vi "Read Live Trav position.vi"() -> ()   [LabVIEW 2021]
uses:
  <vilib>/BioRobotics/Sensor Drivers/OptiTrack Motive/Controls/OptiTrack_Comm Server Data.ctl
  <vilib>/BioRobotics/Sensor Drivers/OptiTrack Motive/Controls/OptiTrack_Parameters.ctl
  <vilib>/BioRobotics/Sensor Drivers/OptiTrack Motive/Controls/OptiTrack_Frame Data.ctl
  <vilib>/BioRobotics/Sensor Drivers/OptiTrack Motive/Controls/OptiTrack_Comm FGV Action.ctl
  <vilib>/Utility/miscctls.llb/LVPointTypeDef.ctl
  ADAM Client/Sub VIs/ADAM Controls/Update_scan_value.ctl
  Optitrack Global.vi
  <vilib>/BioRobotics/Sensor Drivers/OptiTrack Motive/OptiTrack Motive.lvlib
  <vilib>/BioRobotics/Common Tools/BioRobotics Common Tools.lvlib
  <vilib>/Analysis/NI_AALBase.lvlib
panel:
  in  "Teach Position X,Y,Z,":sgl[](array[numeric])
  in  "Set Position to":bool
  in  "Averaging":i32=30
  out "X,Y,Z, Rx, Ry, Rz":sgl[](array[numeric])
  out "OptiTrack Data":T1
  in  "stop":bool
  out "Streaming Server Running":bool
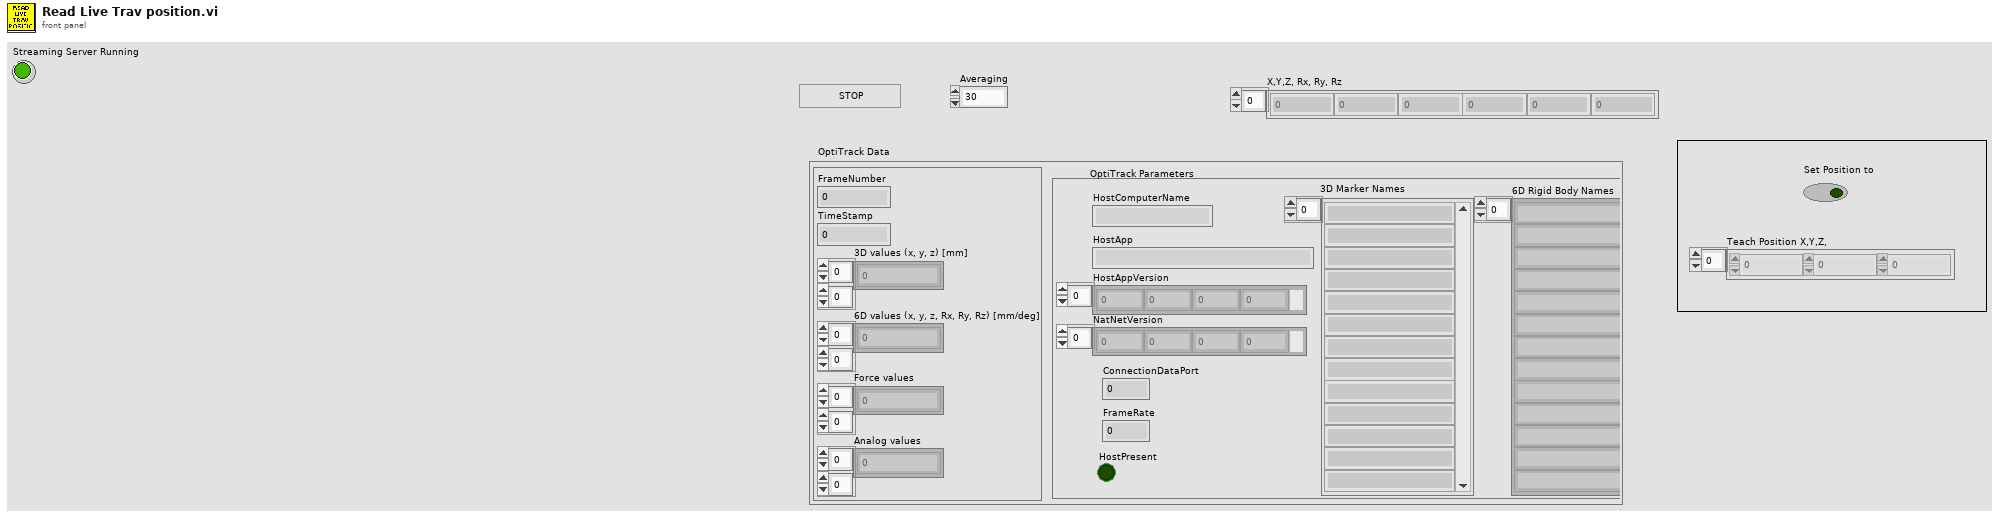
[diagram p1: front panel]
types:
  T1 = typedef "OptiTrack Motive.lvlib/OptiTrack_Comm Server Data.ctl" = cluster{"OptiTrack Parameters":T2, "OptiTrack Frame Data":T3}
  T2 = typedef "OptiTrack Motive.lvlib/OptiTrack_Parameters.ctl" = cluster{"HostComputerName":string, "HostApp":string, "HostAppVersion":u8[], "NatNetVersion":u8[], "ConnectionDataPort":u16, "HostPresent":bool, "3D Marker Names":string[], "6D Rigid Body Names":string[], "Skeletons":string[], "Force Plate Channel Names":string[], "Analog Channel Names":string[], "FrameRate":sgl}
  T3 = typedef "OptiTrack Motive.lvlib/OptiTrack_Frame Data.ctl" = cluster{"FrameNumber":i32, "TimeStamp":i64, "3D values (x, y, z) [mm]":sgl[][], "6D values (x, y, z, Rx, Ry, Rz) [mm/deg]":sgl[][], "Force values":sgl[][], "Analog values":sgl[][]}
  T4 = typedef "LVPointTypeDef.ctl" = cluster{"Horizontal":i16, "Vertical":i16}
  T5 = typedef "OptiTrack Motive.lvlib/OptiTrack_Comm FGV Action.ctl" = enum16{"Initialize", "Set Ethernet Settings", "Read All Data", "Set Parameters", "Start Streaming Server", "Stop Streaming Server", "Set Streaming Data", "Get Streaming Data", "Save Configuration", "Load Configuration", "Connect", "Disconnect", "Streaming Server Running", "Get Data"}
  T6 = typedef "Update_scan_value.ctl" = cluster{"Channel Name":string, "New Value":dbl, "!Auto_Off":bool}
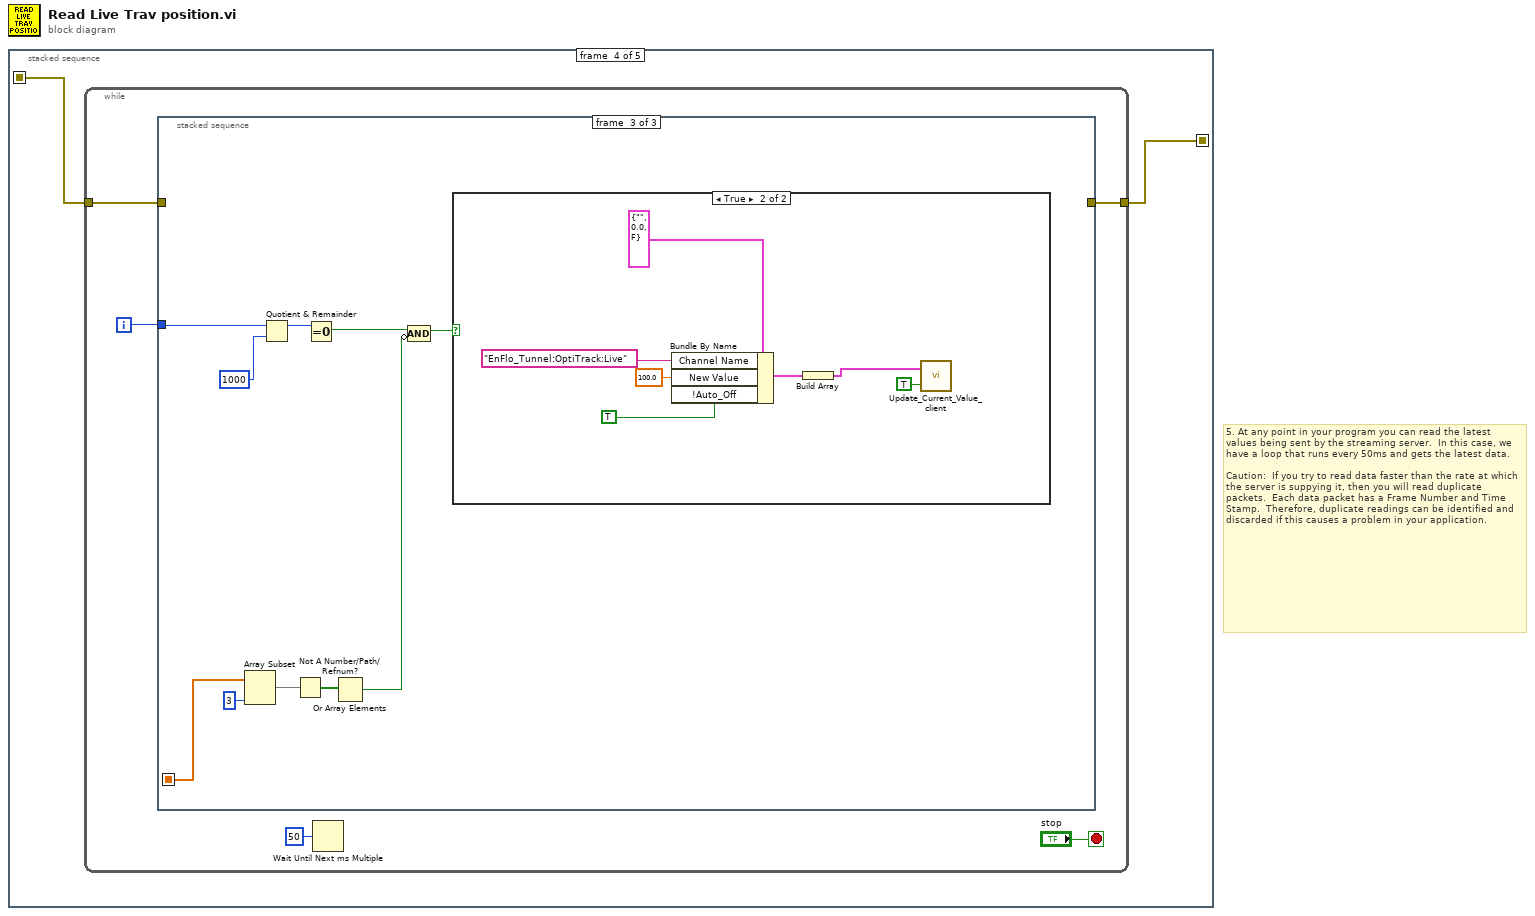
[diagram p0: block diagram]
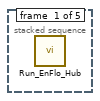
[diagram p2: hidden frame]
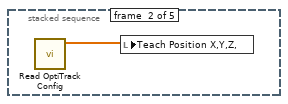
[diagram p3: hidden frame]
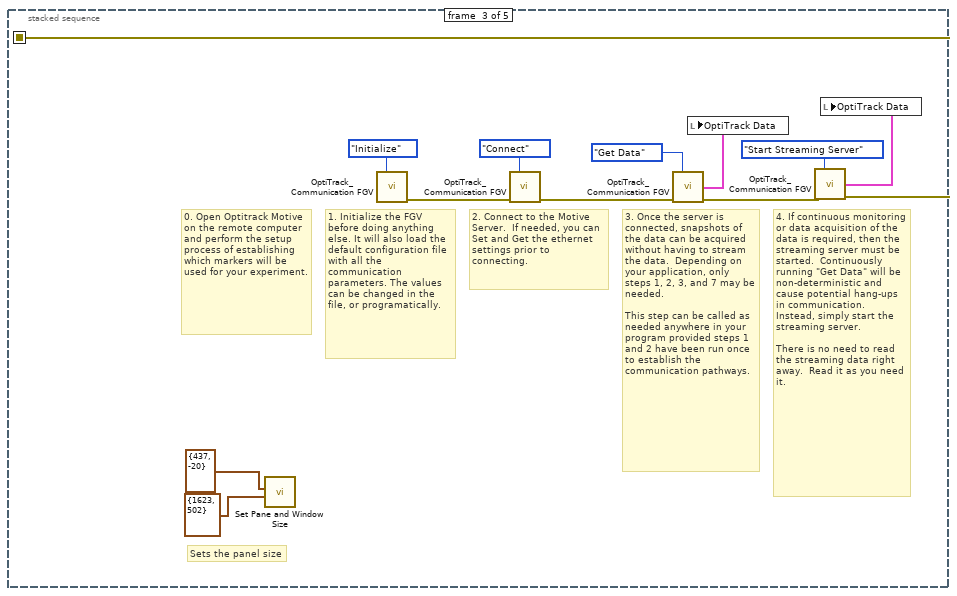
[diagram p4: hidden frame]
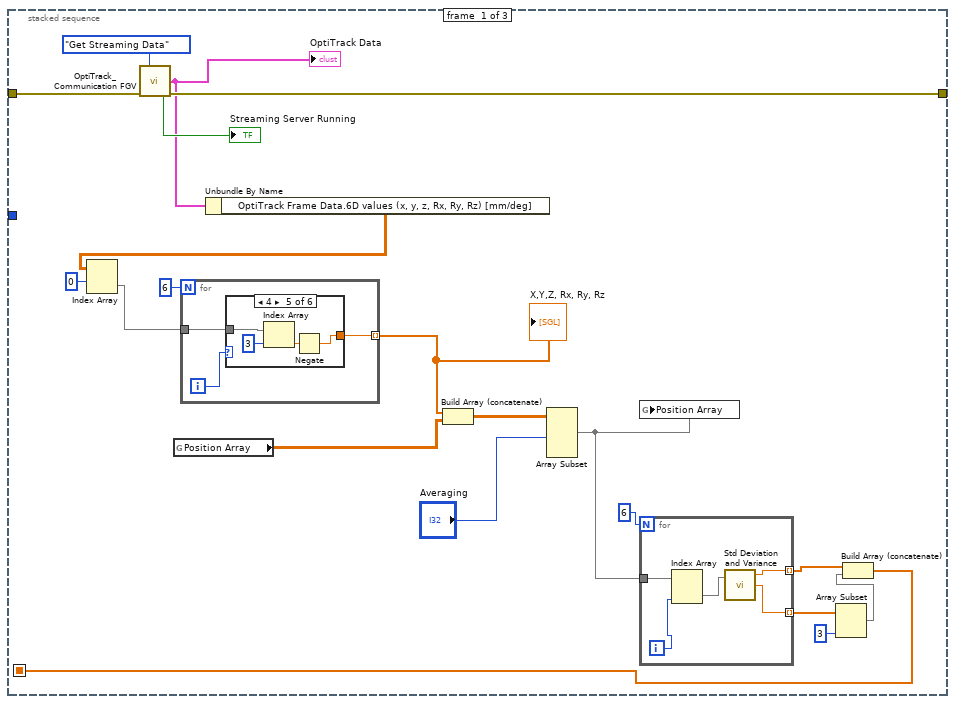
[diagram p5: hidden frame]
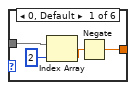
[diagram p6: hidden frame]
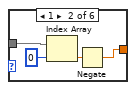
[diagram p7: hidden frame]
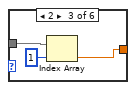
[diagram p8: hidden frame]
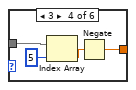
[diagram p9: hidden frame]
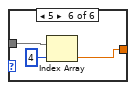
[diagram p10: hidden frame]
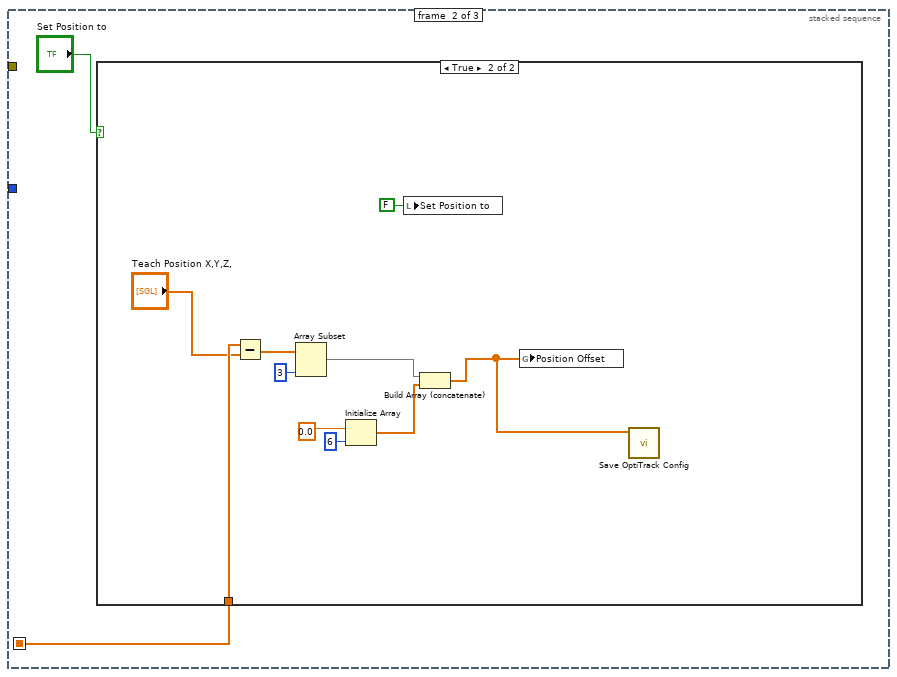
[diagram p11: hidden frame]
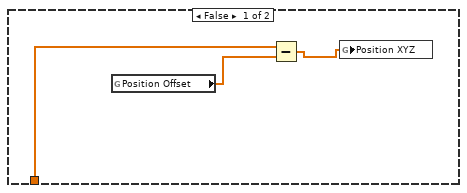
[diagram p12: hidden frame]
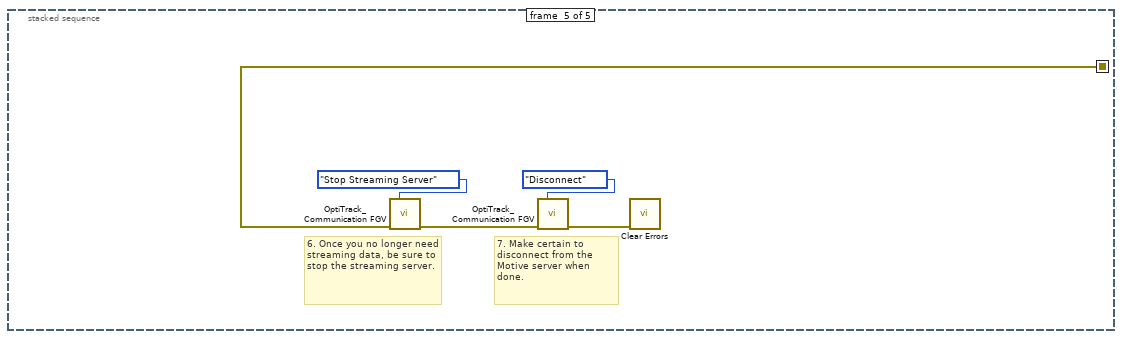
[diagram p14: hidden frame]
diagram:
  # "5. At any point in your program you can read the latest values being sent by the streaming server.  In this case, we have a loop that runs every 50ms and gets the latest data.\n\nCaution:  If you try to read data faster than the rate at which the server is suppying it, then you will read duplicate packets.  Each data packet has a Frame Number and Time Stamp.  Therefore, duplicate readings can be identified and discarded if this causes a problem in your application."
  n1 = stacked-sequence {
    seq-local: [_ _ w2 _ _] -> [_ _ _ w15 _]
    seq-local: [_ _ _ w14 _] -> [_ _ _ _ w103]
    frame #0 {
      n2 = call "Run_EnFlo_Hub.vi"() -> ()  [unwired: 7 in, 1 out]
    }
    frame #1 {
      n3 = call "Read OptiTrack Config.vi"() -> ("Offset Array"=w1:dbl[])  [unwired: 10 in, 1 out]
      n4 = local write "Teach Position X,Y,Z,"(w1) -> ()
    }
    frame #2 {
      # "Sets the panel size"
      # "0. Open Optitrack Motive on the remote computer and perform the setup process of establishing which markers will be used for your experiment."
      # "4. If continuous monitoring or data acquisition of the data is required, then the streaming server must be started.  Continuously running \"Get Data\" will be non-deterministic and cause potential hang-ups in communication.  Instead, simply start the streaming server.\n\nThere is no need to read the streaming data right away.  Read it as you need it."
      # "3. Once the server is connected, snapshots of the data can be acquired without having to stream the data.  Depending on your application, only steps 1, 2, 3, and 7 may be needed.  \n\nThis step can be called as needed anywhere in your program provided steps 1 and 2 have been run once to establish the communication pathways."
      # "2. Connect to the Motive Server.  If needed, you can Set and Get the ethernet settings prior to connecting."
      # "1. Initialize the FGV before doing anything else. It will also load the default configuration file with all the communication parameters. The values can be changed in the file, or programatically."
      n5 = call <vilib>:"Set Pane and Window Size.vi"("Window Size"=T4 {"Horizontal"=1623, "Vertical"=502}, "Pane Origin"=T4 {"Horizontal"=437, "Vertical"=-20}) -> ()  [unwired: 9 in, 1 out]
      n6 = call <vilib>:"OptiTrack_Communication FGV.vi"("OptiTrack Comm FGV Action"=OptiTrack_Comm_FGV_Action."Initialize") -> ("error out"=w11:errorcluster)  [unwired: 9 in, 5 out]
      n7 = call <vilib>:"OptiTrack_Communication FGV.vi"("OptiTrack Comm FGV Action"=OptiTrack_Comm_FGV_Action."Connect", "error in (no error)"=w11) -> ("error out"=w9:errorcluster)  [unwired: 8 in, 5 out]
      n8 = call <vilib>:"OptiTrack_Communication FGV.vi"("OptiTrack Comm FGV Action"=OptiTrack_Comm_FGV_Action."Get Data", "error in (no error)"=w9) -> ("OptiTrack Data"=w8:T1, "error out"=w7:errorcluster)  [unwired: 8 in, 4 out]
      n9 = local write "OptiTrack Data"(w8) -> ()
      n10 = call <vilib>:"OptiTrack_Communication FGV.vi"("OptiTrack Comm FGV Action"=OptiTrack_Comm_FGV_Action."Start Streaming Server", "error in (no error)"=w7) -> ("OptiTrack Data"=w5:T1, "error out"=w2:errorcluster)  [unwired: 8 in, 4 out]
      n11 = local write "OptiTrack Data"(w5) -> ()
    }
    frame #3 {
      n12 = while {
        tunnel: [w18] -> w14
        tunnel: w15 -> [w19]
        i -> [w16]
        stop <- "stop" stop-if-true
        n13 = stacked-sequence {
          seq-local: [w21 _ _] -> [_ w72 w92]
          tunnel: w19 -> [w40 _ _]
          tunnel: [w37 _ _] -> w18
          tunnel: w16 -> [_ _ w95]
          frame #0 {
            n14 = call <vilib>:"OptiTrack_Communication FGV.vi"("OptiTrack Comm FGV Action"=OptiTrack_Comm_FGV_Action."Get Streaming Data", "error in (no error)"=w40) -> ("OptiTrack Data"=w36:T1, "Streaming Server Running"=→"Streaming Server Running":bool, "error out"=w37:errorcluster)  [unwired: 8 in, 3 out]
            "OptiTrack Data" <- w36
            n15 = global read "Optitrack Global.vi" "Position Array"() -> (w33:dbl[][])
            n16 = Unbundle By Name(w36) -> ("OptiTrack Frame Data.6D values (x, y, z, Rx, Ry, Rz) [mm/deg]"=w35:sgl[][])
            n17 = Index Array(array=w35, index (row)=0) -> (element=w28:sgl[])  [unwired: 1 in]
            n18 = for {
              N: 6 -> [_]
              tunnel: w28 -> [w42]
              tunnel: [w41] -> w26 mode=indexing
              i -> [w43]
              n19 = case shown="4" w43 {
                tunnel: w42 -> [w46 w50 w53 w57 w61 w64]
                tunnel: [w44 w48 w52 w55 w59 w63] -> w41
                frame 0, Default {
                  n20 = Index Array(array=w46, index=2) -> (element=w45:sgl)
                  n21 = Negate(x=w45) -> (-x=w44:sgl)
                }
                frame 1 {
                  n22 = Index Array(array=w50, index=0) -> (element=w49:sgl)
                  n23 = Negate(x=w49) -> (-x=w48:sgl)
                }
                frame 2 {
                  n24 = Index Array(array=w53, index=1) -> (element=w52:sgl)
                }
                frame 3 {
                  n25 = Index Array(array=w57, index=5) -> (element=w56:sgl)
                  n26 = Negate(x=w56) -> (-x=w55:sgl)
                }
                frame 4 {
                  n27 = Index Array(array=w61, index=3) -> (element=w60:sgl)
                  n28 = Negate(x=w60) -> (-x=w59:sgl)
                }
                frame 5 {
                  n29 = Index Array(array=w64, index=4) -> (element=w63:sgl)
                }
              }
            }
            "X,Y,Z, Rx, Ry, Rz" <- w26
            n30 = Build Array (concatenate)(w26, w33) -> (w32:dbl[][])
            n31 = Array Subset(array=w32, length (row)="Averaging") -> (w29:dbl[][])  [unwired: 3 in]
            n32 = global write "Optitrack Global.vi" "Position Array"(w29) -> ()
            n33 = for {
              N: 6 -> [_]
              tunnel: w29 -> [w70]
              tunnel: [w67] -> w25 mode=indexing
              tunnel: [w66] -> w24 mode=indexing
              i -> [w69]
              n34 = Index Array(array=w70, index (col)=w69) -> (element=w68:dbl[])  [unwired: 1 in]
              n35 = call <vilib>:"Std Deviation and Variance.vi"("X"=w68) -> ("mean"=w67:dbl, "standard deviation"=w66:dbl)  [unwired: 1 in, 1 out]
            }
            n36 = Array Subset(array=w24, length=3) -> (w22:dbl[])  [unwired: 1 in]
            n37 = Build Array (concatenate)(w25, w22) -> (w21:dbl[])
          }
          frame #1 {
            n38 = case shown="True" "Set Position to" {
              tunnel: w72 -> [w74 w85]
              frame False {
                n39 = global read "Optitrack Global.vi" "Position Offset"() -> (w75:dbl[])
                n40 = Subtract(x=w74, y=w75) -> (x-y=w73:dbl[])
                n41 = global write "Optitrack Global.vi" "Position XYZ"(w73) -> ()
              }
              frame True {
                n42 = Subtract(x=w85, y="Teach Position X,Y,Z,") -> (x-y=w83:dbl[])
                n43 = Array Subset(array=w83, length=3) -> (w81:dbl[])  [unwired: 1 in]
                n44 = Initialize Array(0.0, 6 ("dimension size")) -> (w77:dbl[])
                n45 = local write "Set Position to"(FALSE ("Set Position to")) -> ()
                n46 = Build Array (concatenate)(w81, w77) -> (w76:dbl[])
                n47 = global write "Optitrack Global.vi" "Position Offset"(w76) -> ()
                n48 = call "Save OptiTrack Config.vi"("Offset Array"=w76) -> ()  [unwired: 10 in, 1 out]
              }
            }
          }
          frame #2 {
            n49 = Array Subset(array=w92, length=3) -> (w90:dbl[])  [unwired: 1 in]
            n50 = Quotient & Remainder(x=w95, y=1000) -> (x-y*floor(x/y)=w93:i32)  [unwired: 1 out]
            n51 = Not A Number/Path/Refnum?(number/path/refnum=w90) -> (NaN/Path/Refnum?=w89:bool[])
            n52 = Equal To 0?(x=w93) -> (x = 0?=w88:bool)
            n53 = Or Array Elements(Boolean array=w89) -> (logical OR=w86:bool)
            n54 = Compound Arithmetic op=AND(w88, invert w86) -> (w87:bool)
            n55 = case shown="True" w87 {
              frame False {
              }
              frame True {
                n56 = Bundle By Name(cluster=T6 {"Channel Name"="", "New Value"=0.0, "!Auto_Off"=FALSE} ("Update Scan Value Cluster"), "Channel Name"="EnFlo_Tunnel:OptiTrack:Live", "New Value"=100.0, "!Auto_Off"=TRUE) -> (w98:T6)
                n57 = Build Array(w98) -> (w97:T6[])
                n58 = call "Update_Current_Value_client.vi"("Don't Bother with check?"=TRUE, "Update array in"=w97) -> ()
              }
            }
          }
        }
        n59 = Wait Until Next ms Multiple(millisecond multiple=u32 50) -> ()  [unwired: 1 out]
      }
    }
    frame #4 {
      # "7. Make certain to disconnect from the Motive server when done."
      # "6. Once you no longer need streaming data, be sure to stop the streaming server."
      n60 = call <vilib>:"OptiTrack_Communication FGV.vi"("OptiTrack Comm FGV Action"=OptiTrack_Comm_FGV_Action."Stop Streaming Server", "error in (no error)"=w103) -> ("error out"=w106:errorcluster)  [unwired: 8 in, 5 out]
      n61 = call <vilib>:"OptiTrack_Communication FGV.vi"("OptiTrack Comm FGV Action"=OptiTrack_Comm_FGV_Action."Disconnect", "error in (no error)"=w106) -> ("error out"=w107:errorcluster)  [unwired: 8 in, 5 out]
      n62 = call <vilib>:"Clear Errors.vi"("error in (no error)"=w107) -> ()  [unwired: 5 in, 2 out]
    }
  }
